vi "Slope Calibration.vi"() -> ()   [LabVIEW 2013]
panel:
  in  "Record Slope":bool
  in  "Gather Data":bool
  out "Slope (nm/V)":dbl
  out "XY Graph":cluster{"X":dbl[], "Y":dbl[]}(graph)
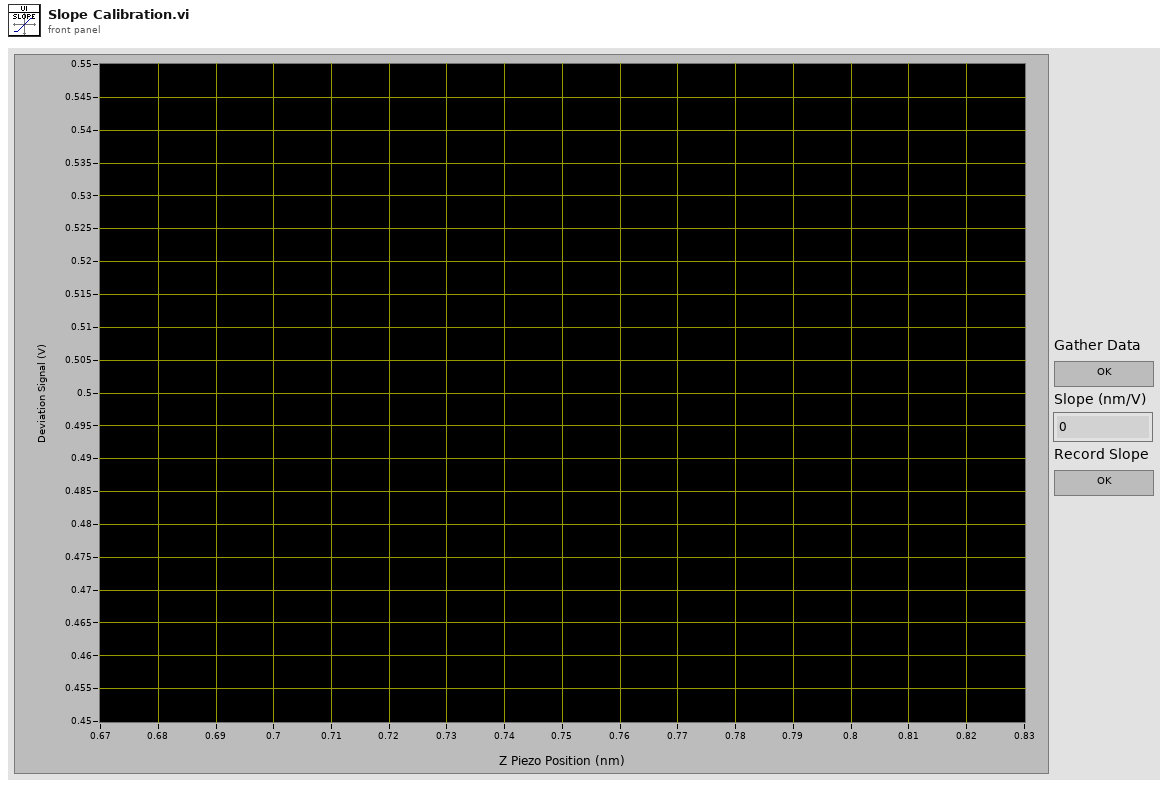
[diagram p1: front panel]
types:
  T1 = typedef "LVCursorListTypeDef.ctl" = cluster{"Name":string, "Color":u32, "Style":u8, "Point Style":u8, "Name Visible":bool, "Allow Drag":bool, "Cursor Mode":u32, "Plot":i32, "Index":i32, "Position":cluster{"X":dbl, "Y":dbl}, "X Scale":u32, "Y Scale":u32, "Watch Plots":i32[], "Watch All Plots":bool, "Plot Area":i32, "Label Offset":cluster{"X":dbl, "Y":dbl}}[]
  T2 = cluster{"Name":string, "Color":u32, "Style":u8, "Point Style":u8, "Name Visible":bool, "Allow Drag":bool, "Cursor Mode":u32, "Plot":i32, "Index":i32, "Position":cluster{"X":dbl, "Y":dbl}, "X Scale":u32, "Y Scale":u32, "Watch Plots":i32[], "Watch All Plots":bool, "Plot Area":i32, "Label Offset":cluster{"X":dbl, "Y":dbl}}
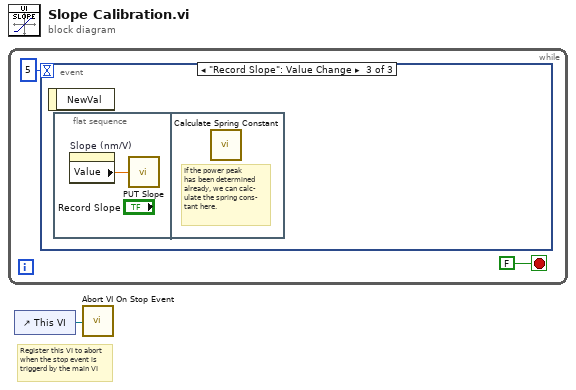
[diagram p0: block diagram]
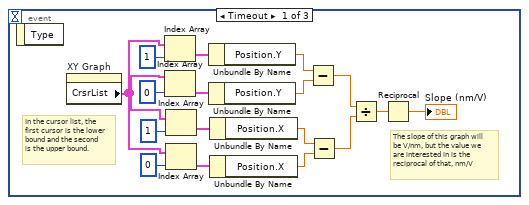
[diagram p2: hidden frame]
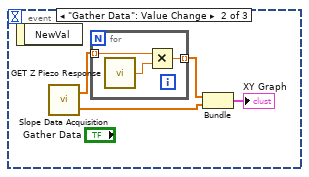
[diagram p3: hidden frame]
diagram:
  # "Register this VI to abort\nwhen the stop event is\ntriggerd by the main VI"
  n1 = while {
    stop <- FALSE stop-if-true
    n2 = event shown="[2] \"Record Slope\": Value Change" {
      selector: _ -> [_ _ _]
      dyn-events: _ -> [_ _ _]
      timeout: 5 -> [_ _ _]
      event Timeout {
        # "The slope of this graph will\nbe V/nm, but the value we\nare interested in is the \nreciprocal of that, nm/V"
        # "In the cursor list, the\nfirst cursor is the lower\nbound and the second \nis the upper bound."
        n3 = event-data() -> ()  [unwired: 1 in, 1 out]
        n4 = property on="XY Graph" class="XYGraph (strict)"() -> ("CrsrList"=w8:T1)  [unwired: 2 in, 2 out]
        n5 = Index Array(array=w8, index=1) -> (element=w18:T2)
        n6 = Index Array(array=w8, index=0) -> (element=w17:T2)
        n7 = Index Array(array=w8, index=1) -> (element=w11:T2)
        n8 = Index Array(array=w8, index=0) -> (element=w12:T2)
        n9 = Unbundle By Name(w18) -> ("Position.Y"=w16:dbl)
        n10 = Unbundle By Name(w17) -> ("Position.Y"=w15:dbl)
        n11 = Unbundle By Name(w11) -> ("Position.X"=w13:dbl)
        n12 = Unbundle By Name(w12) -> ("Position.X"=w14:dbl)
        n13 = Subtract(x=w16, y=w15) -> (x-y=w7:dbl)
        n14 = Subtract(x=w13, y=w14) -> (x-y=w6:dbl)
        n15 = Divide(x=w7, y=w6) -> (x/y=w5:dbl)
        n16 = Reciprocal(x=w5) -> (1/x=→"Slope (nm/V)":dbl)
      }
      event "Gather Data": Value Change {
        n17 = event-data() -> ()  [unwired: 1 in, 1 out]
        n18 = call "Slope Data Acquisition.vi"() -> ("Deviation Signal"=w22:dbl[], "Z Piezo Signal"=w24:dbl[])
        n19 = for {
          tunnel: w24 -> [w27] mode=indexing
          tunnel: [w25] -> w23 mode=indexing
          n20 = call "GET Z Piezo Response.vi"() -> ("Z Piezo Response"=w26:dbl)
          n21 = Multiply(x=w27, y=w26) -> (x*y=w25:dbl)
        }
        n22 = Bundle(w23, "Deviation Signal"=w22) -> (→"XY Graph":cluster{dbl[], "Deviation Signal":dbl[]})  [unwired: 1 in]
      }
      event "Record Slope": Value Change {
        n23 = event-data() -> ()  [unwired: 1 in, 1 out]
        n24 = flat-sequence {
          frame #0 {
            n25 = property on="Slope (nm/V)" class="DigNum (strict)"() -> ("Value"=w28:dbl)  [unwired: 2 in, 2 out]
            n26 = call "PUT Slope.vi"("Slope"=w28) -> ()
          }
          frame #1 {
            # "If the power peak\nhas been determined\nalready, we can calc-\nulate the spring cons-\ntant here."
            n27 = call "Calculate Spring Constant.vi"() -> ()  [unwired: 1 in]
          }
        }
      }
    }
  }
  n28 = control-ref of="This VI"() -> (w1:refnum<vi>)
  n29 = call "Abort VI On Stop Event.vi"("VI Reference"=w1) -> ()
